vi "Using a previously exported configuration.vi"(8 "error in (no error)":errorcluster, 9 "export file path":path, 10 "target in":refnum<k24>, 11 "configuration file path":path) -> (0 "error out":errorcluster)   [LabVIEW 2019]
uses:
  NationalInstruments.VeriStand.SystemDefinitionAPI
  <vilib>/addons/VeriStand Custom Device Scripting APIs/Instrument Addon/API/TypeDefs/Message Settings.ctl
  <vilib>/addons/VeriStand Custom Device Scripting APIs/Instrument Addon/API/TypeDefs/Protection Types.ctl
  <vilib>/addons/VeriStand Custom Device Scripting APIs/Instrument Addon/API/TypeDefs/Single Channel Format Settings.ctl
  <vilib>/addons/VeriStand Custom Device Scripting APIs/Instrument Addon/API/TypeDefs/Command Settings.ctl
  <vilib>/NI VeriStand/Custom Device API/Custom Device Item Ref.ctl
  <vilib>/addons/VeriStand Custom Device Scripting APIs/Instrument Addon/API/TypeDefs/Padding.ctl
  <vilib>/addons/VeriStand Custom Device Scripting APIs/Instrument Addon/API/TypeDefs/Array Type Cast Settings.ctl
  <vilib>/addons/VeriStand Custom Device Scripting APIs/Instrument Addon/API/TypeDefs/Array Element.ctl
  <vilib>/addons/VeriStand Custom Device Scripting APIs/Instrument Addon/Shared Directory/Type Cast Type.ctl
  <vilib>/addons/VeriStand Custom Device Scripting APIs/Instrument Addon/Shared Directory/Endian.ctl
  <vilib>/addons/VeriStand Custom Device Scripting APIs/Instrument Addon/API/Channels/Create Global MetaData Channel - Array - Type Cast.vi
  <vilib>/addons/VeriStand Custom Device Scripting APIs/Instrument Addon/API/Messages/Create Message - Value Change & Trigger.vi
  <vilib>/addons/VeriStand Custom Device Scripting APIs/Instrument Addon/API/Channels/Create MetaData Channel - Single Channel - Format.vi
  <vilib>/addons/VeriStand Custom Device Scripting APIs/Instrument Addon/API/Instrument Addon Scripting API.lvlib
  <vilib>/NI VeriStand/Custom Device API/Custom Device API.lvlib
  <vilib>/addons/VeriStand Custom Device Scripting APIs/Instrument Addon/Shared Directory/Instrument Addon Shared.lvlib
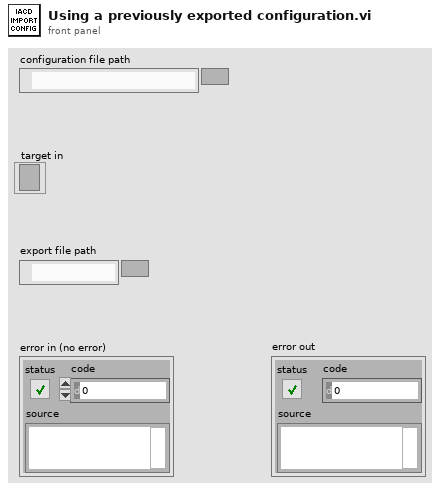
[diagram p1: front panel]
types:
  T1 = typedef "Custom Device API.lvlib/Custom Device Item Ref.ctl" = u64
  T2 = cluster{"Variable Name":string, "Channel Ref in":T1}
  T3 = typedef "Instrument Addon Scripting API.lvlib/Array Type Cast Settings.ctl" = cluster{"Elements":T4[], "Delimiter":string, "Type":T5, "Endian":T6}
  T4 = typedef "Instrument Addon Scripting API.lvlib/Array Element.ctl" = cluster{"Name":string, "Default Value":dbl, "Units":string}
  T5 = typedef "Instrument Addon Shared.lvlib/Type Cast Type.ctl" = enum16{"DBL", "SGL", "U64", "U32", "U16", "U8", "I64", "I32", "I16", "I8"}
  T6 = typedef "Instrument Addon Shared.lvlib/Endian.ctl" = enum16{"Native", "Little", "Big"}
  T7 = typedef "Instrument Addon Scripting API.lvlib/Padding.ctl" = cluster{"Pad Value":u8, "Length":u32}
  T8 = typedef "Instrument Addon Scripting API.lvlib/Command Settings.ctl" = cluster{"Command Format":string, "Linked Channels":cluster{"Variable Name":string, "Channel Ref in":T1}[], "Use Padding?":bool, "Padding":T7}
  T9 = typedef "Instrument Addon Scripting API.lvlib/Single Channel Format Settings.ctl" = cluster{"Format String":string, "Default Value":dbl, "Units":string}
  T10 = typedef "Instrument Addon Scripting API.lvlib/Message Settings.ctl" = cluster{"Protection":T11, "Enable Periodic Default":bool, "Trigger Channel refnum":u64}
  T11 = typedef "Instrument Addon Scripting API.lvlib/Protection Types.ctl" = enum16{"None", "CRC-32", "Checksum U16", "Checksum U32", "Checksum U8"}
  T12 = cluster{"Variable Name":string, "Channel Ref in":T1}[]
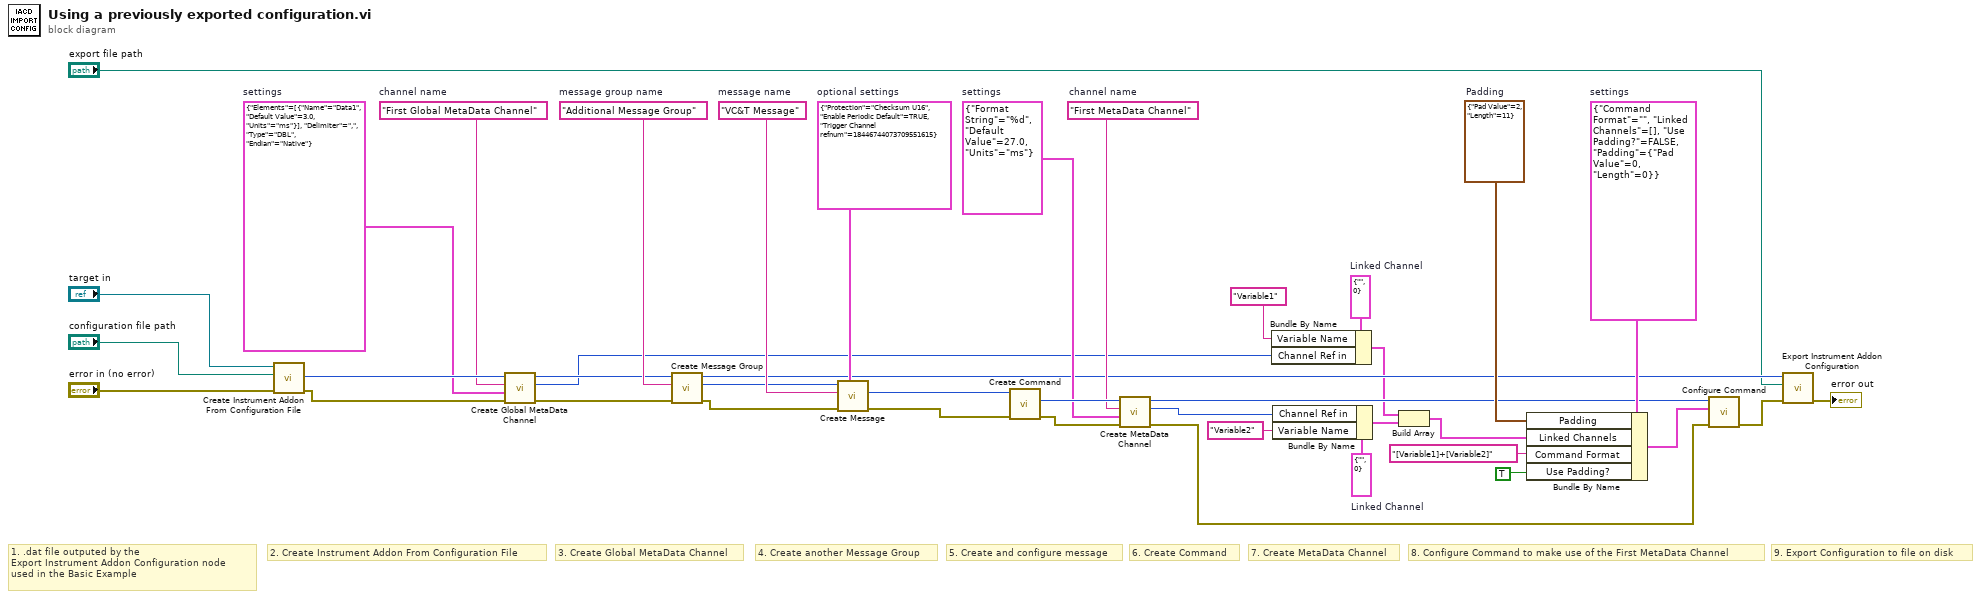
[diagram p0: block diagram]
diagram:
  w4 = T2 {"Variable Name"="", "Channel Ref in"=0}  # Linked Channel
  w6 = T3 {"Elements"=[{"Name"="Data1", "Default Value"=3.0, "Units"="ms"}], "Delimiter"=",", "Type"=enum."DBL", "Endian"=enum."Native"}  # settings
  w7 = "First Global MetaData Channel"  # channel name
  w20 = T7 {"Pad Value"=2, "Length"=11}  # Padding
  w26 = T2 {"Variable Name"="", "Channel Ref in"=0}  # Linked Channel
  w28 = T8 {"Command Format"="", "Linked Channels"=[], "Use Padding?"=FALSE, "Padding"={"Pad Value"=0, "Length"=0}}  # settings
  w30 = T9 {"Format String"="%d", "Default Value"=27.0, "Units"="ms"}  # settings
  w31 = "First MetaData Channel"  # channel name
  w34 = T10 {"Protection"=enum."Checksum U16", "Enable Periodic Default"=TRUE, "Trigger Channel refnum"=18446744073709551615}  # optional settings
  w36 = "VC&T Message"  # message name
  w37 = "Additional Message Group"  # message group name
  # "3. Create Global MetaData Channel"
  # "9. Export Configuration to file on disk"
  # "8. Configure Command to make use of the First MetaData Channel"
  # "7. Create MetaData Channel"
  # "6. Create Command"
  # "5. Create and configure message"
  # "4. Create another Message Group"
  # "2. Create Instrument Addon From Configuration File"
  # "1. .dat file outputed by the \nExport Instrument Addon Configuration node \nused in the Basic Example"
  n1 = call <vilib>:"Create Instrument Addon From Configuration File.vi"("error in (no error)"="error in (no error)", "configuration file path"="configuration file path", "target in"="target in") -> ("error out"=w9:errorcluster, "instrument addon refnum"=w11:T1)  [unwired: 6 in, 1 out]
  n2 = call-poly <vilib>:"Create Global MetaData Channel.vi"("error in (no error)"=w9, "settings"=w6, "channel name"=w7, "instrument addon refnum in"=w11) -> ("error out"=w8:errorcluster, "array refnum"=w1:T1, "instrument addon refnum out"=w10:T1)  [unwired: 4 in, 1 out]
  n3 = call <vilib>:"Create Message Group.vi"("error in (no error)"=w8, "message group name"=w37, "instrument addon refnum in"=w10) -> ("error out"=w33:errorcluster, "message group refnum out"=w35:T1, "instrument addon refnum out"=w14:T1)  [unwired: 6 in]
  n4 = call-poly <vilib>:"Create Message.vi"("optional settings"=w34, "error in (no error)"=w33, "message name"=w36, "message group refnum in"=w35) -> ("error out"=w19:errorcluster, "message refnum out"=w18:T1)  [unwired: 5 in, 1 out]
  n5 = call <vilib>:"Create Command.vi"("error in"=w19, "message refnum In"=w18) -> ("error out"=w29:errorcluster, "command refnum"=w32:T1)  [unwired: 7 in, 1 out]
  n6 = call-poly <vilib>:"Create MetaData Channel.vi"("error in (no error)"=w29, "settings"=w30, "channel name"=w31, "command refnum in"=w32) -> ("error out"=w15:errorcluster, "channel refnum"=w22:T1, "command refnum out"=w17:T1)  [unwired: 5 in]
  n7 = Bundle By Name(cluster=w4, "Variable Name"="Variable1", "Channel Ref in"=w1) -> (w2:T2)
  n8 = Bundle By Name(cluster=w26, "Channel Ref in"=w22, "Variable Name"="Variable2") -> (w24:T2)
  n9 = Build Array(w2, w24) -> (w23:T12)
  n10 = Bundle By Name(cluster=w28, "Padding"=w20, "Linked Channels"=w23, "Command Format"="[Variable1]+[Variable2]", "Use Padding?"=TRUE) -> (w16:T8)
  n11 = call <vilib>:"Configure Command.vi"("error in (no error)"=w15, "settings"=w16, "command refnum in"=w17) -> ("error out"=w13:errorcluster)  [unwired: 7 in, 1 out]
  n12 = call <vilib>:"Export Instrument Addon Configuration.vi"("error in (no error)"=w13, "export file path"="export file path", "instrument addon refnum in"=w14) -> ("error out"=→"error out":errorcluster)  [unwired: 7 in, 1 out]
